vi "Fast Holo2 SLM.vi"   [LabVIEW 2014]
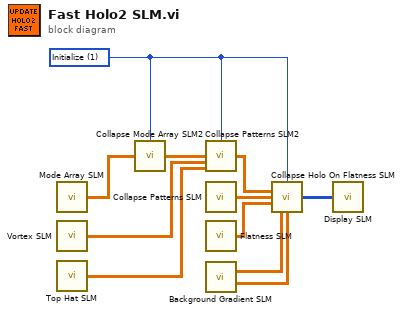
[diagram p0: block diagram]
diagram:
  w3 = u16 1 items=["Read", "Initialize"] ("Action")
  n1 = call "Mode Array SLM.vi"() -> ("mode array"=w4:dbl[][][])  [unwired: 15 in]
  n2 = call "Vortex SLM.vi"() -> ("Vortex"=w6:dbl[][])  [unwired: 15 in]
  n3 = call "Top Hat SLM.vi"() -> ("Top hat"=w5:dbl[][])  [unwired: 15 in]
  n4 = call "Collapse Mode Array SLM2.vi"("Action"=w3, "mode array"=w4) -> ("collapsed mode array"=w7:dbl[][])  [unwired: 13 in]
  n5 = call "Collapse Patterns SLM2.vi"("Action"=w3, "collapsed mode array"=w7, "Vortex"=w6, "Top hat"=w5) -> ("collapsed patterns"=w8:dbl[][])  [unwired: 11 in]
  n6 = call "Collapse Patterns SLM.vi"() -> ("collapsed patterns"=w9:dbl[][])  [unwired: 15 in]
  n7 = call "Flatness SLM.vi"() -> ("flatness"=w10:dbl[][])  [unwired: 15 in]
  n8 = call "Background Gradient SLM.vi"() -> ("gradient"=w2:dbl[][], "holo mask"=w1:dbl[][])  [unwired: 14 in]
  n9 = call "Collapse Holo On Flatness SLM.vi"("Action"=w3, "collapsed patterns 2"=w8, "collapsed patterns"=w9, "flatness"=w10, "gradient"=w2, "holo mask"=w1) -> ("displayed matrix"=w11:u8[][])  [unwired: 9 in]
  n10 = call "Display SLM.vi"("displayed matrix"=w11) -> ()  [unwired: 14 in, 1 out]
